vi "Locate Table.vi"(8 "error in":errorcluster, 11 "picture":refnum<vi>) -> (0 "error out":errorcluster, 3 "T":T1 format="%.3f", 5 "picture":picture)   [LabVIEW 2013]
uses:
  <vilib>/Analysis/Matrix/Datatypes/RealMatrix.ctl
  ROS/Code/SubVIs/BaxterSide.ctl
  <vilib>/Analysis/baseanly.llb/Mean (DBL).vi
  Baxter Examples/Arm Globals.vi
  Move/Move XYZOAT.vi
  Move/Move Axis.vi
  <vilib>/Analysis/baseanly.llb/Real Inverse Matrix.vi
  Prim/Fwd Kenimatics - array.vi
  <vilib>/Analysis/Matrix/Numeric/Multiply/Multiply - RM,RM.vi
  <vilib>/Analysis/Matrix/NI_Matrix.lvlib
  <vilib>/Analysis/NI_AALBase.lvlib
panel:
  out "Range":dbl
  out "result":cluster{"x":dbl, "y":dbl, "a":dbl}
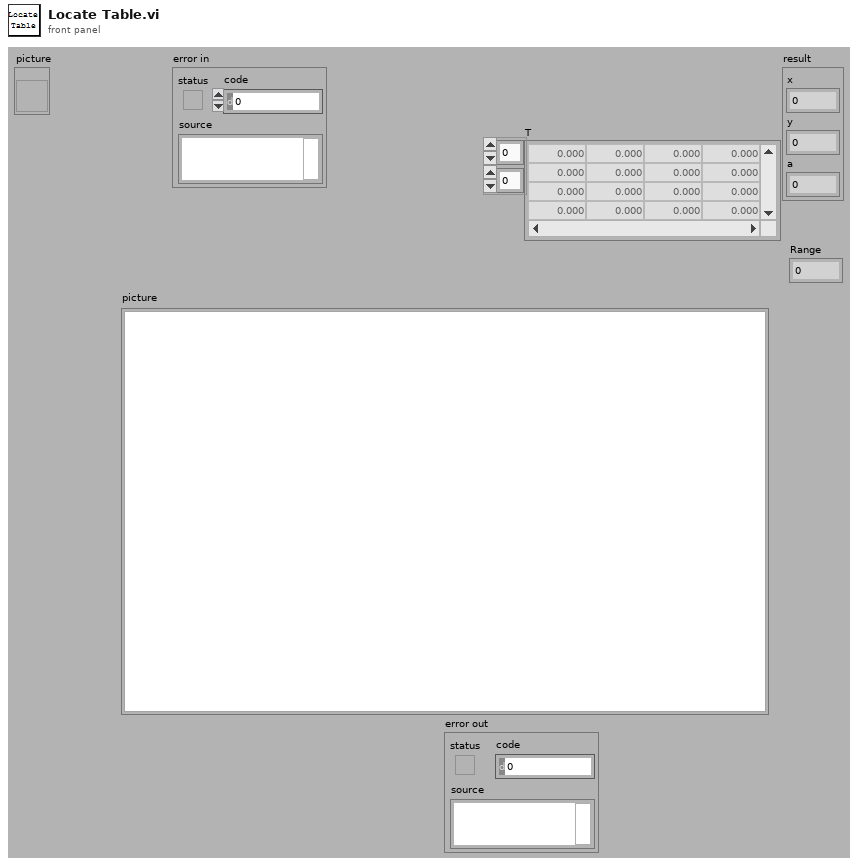
[diagram p1: front panel]
types:
  T1 = typedef "NI_Matrix.lvlib/RealMatrix.ctl" = dbl[][]
  T2 = typedef "BaxterSide.ctl" = enum16{"left", "right"}
  T3 = cluster{"Label":string, "Joints":dbl[], "T":T1}[]
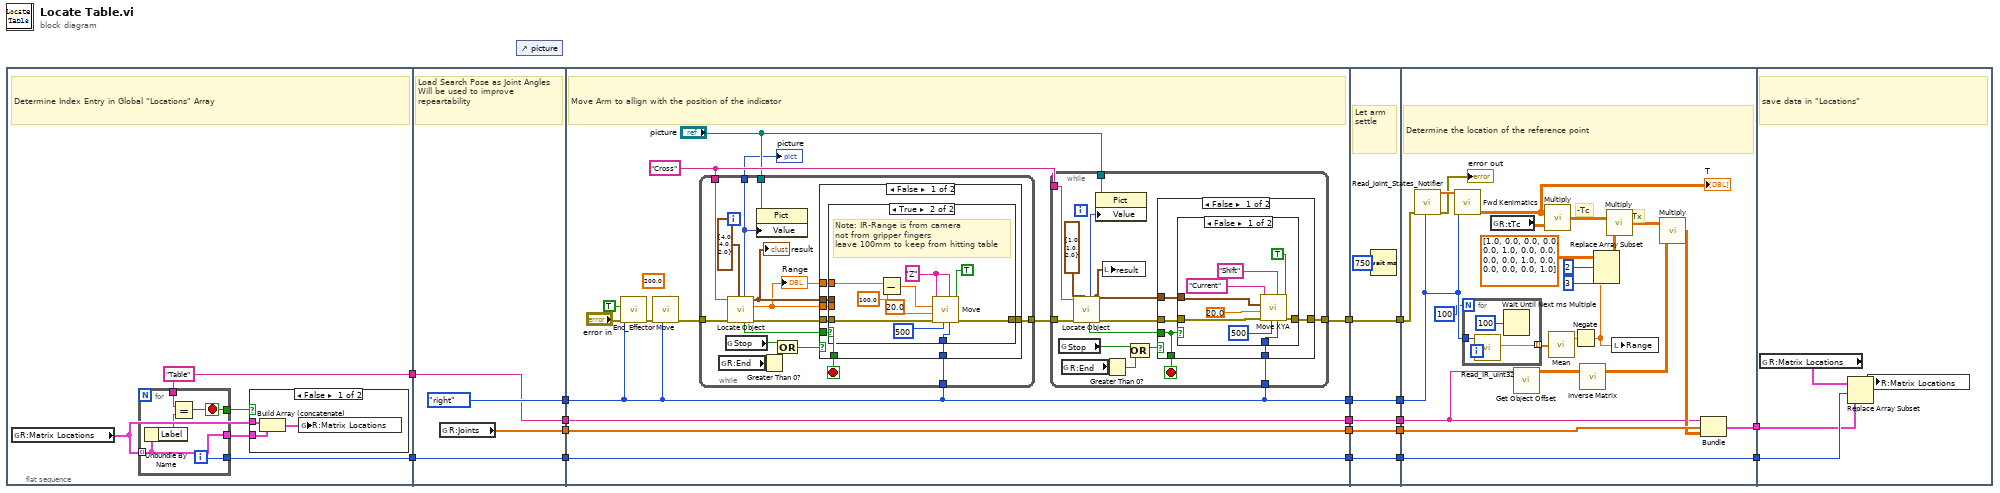
[diagram p0: block diagram]
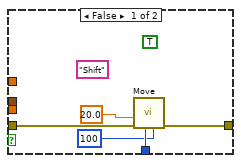
[diagram p5: hidden frame]
diagram:
  n1 = flat-sequence {
    tunnel: [w21] -> w11
    tunnel: [w23] -> w6
    tunnel: [BaxterSide."right" ("Side")] -> w14
    tunnel: [w32] -> w13
    tunnel: [w34] -> w12
    tunnel: w11 -> [w34]
    tunnel: [w33] -> w7
    tunnel: w6 -> [w33]
    tunnel: [w40] -> w17
    tunnel: [w42] -> w15
    tunnel: w14 -> [w40]
    tunnel: w13 -> [w38]
    tunnel: w12 -> [w37]
    tunnel: [w38] -> w10
    tunnel: [w37] -> w9
    tunnel: [w36] -> w8
    tunnel: w7 -> [w36]
    tunnel: [w125] -> w18
    tunnel: w17 -> [w125]
    tunnel: [w124] -> w16
    tunnel: w15 -> [w124]
    tunnel: w10 -> [w122]
    tunnel: w9 -> [w121]
    tunnel: w8 -> [w123]
    tunnel: [w123] -> w5
    tunnel: [w122] -> w4
    tunnel: [w121] -> w2
    tunnel: w18 -> [w139]
    tunnel: w16 -> [w147]
    tunnel: w5 -> [w131]
    tunnel: w4 -> [w134]
    tunnel: [w135] -> w3
    tunnel: w2 -> [w135]
    tunnel: [w132] -> w1
    tunnel: w3 -> [w154]
    tunnel: w1 -> [w153]
    frame #0 {
      w23 = "Table"
      # "Determine Index Entry in Global \"Locations\" Array"
      n2 = global read "Arm Globals.vi" "R:Matrix Locations"() -> (w19:T3)
      n3 = for {
        tunnel: w19 -> [w27] mode=indexing
        tunnel: w23 -> [w31]
        tunnel: [w30] -> w21
        tunnel: [w29] -> w22
        tunnel: [w27] -> w20
        i -> [w30]
        stop <- w29 stop-if-true
        n4 = Unbundle By Name(w27) -> ("Label"=w28:string)
        n5 = Equal?(x=w31, y=w28) -> (x = y?=w29:bool)
      }
      n6 = case shown="False" w22 {
        tunnel: w20 -> [w26 _]
        tunnel: w19 -> [w24 _]
        frame False {
          n7 = Build Array (concatenate)(w24, w26) -> (w25:T3)
          n8 = global write "Arm Globals.vi" "R:Matrix Locations"(w25) -> ()
        }
        frame True {
        }
      }
    }
    frame #1 {
      # "Load Search Pose as Joint Angles\nWill be used to improve repeartability"
      n9 = global read "Arm Globals.vi" "R:Joints"() -> (w32:dbl[])
    }
    frame #2 {
      (unwired) 200.0 ("Z")
      w44 = "Cross"
      # "Move Arm to allign with the position of the indicator"
      n10 = call "End_Effector.vi"("error in"="error in", "Close"=TRUE, "Side"=w40) -> ("error out"=w46:errorcluster)  [unwired: 5 in]
      n11 = call-poly "Move.vi"("Wait Time"=w40, "error in"=w46) -> ("error out"=w45:errorcluster)  [unwired: 9 in]
      n12 = while {
        tunnel: w45 -> [w96]
        tunnel: [w94] -> w48
        tunnel: w44 -> [w91]
        tunnel: w40 -> [w90]
        tunnel: "picture" -> [w85]
        tunnel: [w83] -> w39
        stop <- w88 stop-if-true
        n13 = global read "Arm Globals.vi" "R:End"() -> (w86:i32)
        n14 = global read "Arm Globals.vi" "Stop"() -> (w92:bool)
        n15 = call "Locate Object.vi"("Tolerance"=cluster{"x":dbl, "y":dbl, "a":dbl} {"x"=4.0, "y"=4.0, "a"=2.0}, "error in"=w96, "Object"=w91) -> ("error out"=w95:errorcluster, "Range"=w82:dbl, "result"=w93:cluster{"x":dbl, "y":dbl, "a":dbl}, "Close"=w87:bool, "picture"=w83:picture)  [unwired: 3 in, 1 out]
        "result" <- w93
        "Range" <- w82
        n16 = property class="Pict"(reference=w85, "Value"=w83) -> ()  [unwired: 1 in, 2 out]
        n17 = Greater Than 0?(x=w86) -> (x > 0?=w81:bool)
        n18 = Compound Arithmetic op=OR(w92, w81) -> (w89:bool)
        n19 = case shown="False" w89 {
          selector: w89 -> [_ w119]
          tunnel: w95 -> [w103 w120]
          tunnel: [w102 w120] -> w94
          tunnel: w93 -> [w101 _]
          tunnel: w90 -> [w100 _]
          tunnel: [w99 w119] -> w88
          tunnel: w87 -> [w99 _]
          tunnel: w82 -> [w98 _]
          tunnel: w82 -> [w97 _]
          frame False {
            n20 = case shown="True" w99 {
              tunnel: w103 -> [w108 w118]
              tunnel: [w107 w117] -> w102
              tunnel: w101 -> [_ _]
              tunnel: w100 -> [w106 w109]
              tunnel: w98 -> [_ _]
              tunnel: w97 -> [_ w115]
              frame False {
                (unwired) "Shift" ("Label")
                (unwired) TRUE ("Make Vertical")
                n21 = call-poly "Move.vi"("Side"=100 ("wait time"), "Wait Time"=w106, "error in"=w108, "Speed (mm/s)"=20.0) -> ("error out"=w107:errorcluster)  [unwired: 7 in]
              }
              frame True {
                w112 = "Z" ("Label")
                # "Note: IR-Range is from camera \nnot from gripper fingers\nleave 100mm to keep from hitting table"
                n22 = Subtract(x=w115, y=100.0) -> (x-y=w111:dbl)
                n23 = call-poly "Move.vi"("Make Vertical"=TRUE, "Side"=w109, "Label"=w112, "Wait Time"=500 ("wait time"), "error in"=w118, "Speed"=20.0, "Value"=w111, "Location"=w112) -> ("error out"=w117:errorcluster)  [unwired: 3 in]
              }
            }
          }
          frame True {
          }
        }
      }
      "picture" <- w39
      n24 = while {
        tunnel: w48 -> [w63]
        tunnel: [w61] -> w42
        tunnel: w44 -> [w58]
        tunnel: w40 -> [w57]
        tunnel: "picture" -> [w52]
        stop <- w54 stop-if-true
        n25 = global read "Arm Globals.vi" "Stop"() -> (w59:bool)
        n26 = global read "Arm Globals.vi" "R:End"() -> (w53:i32)
        n27 = call "Locate Object.vi"("Tolerance"=cluster{"x":dbl, "y":dbl, "a":dbl} {"x"=1.0, "y"=1.0, "a"=2.0}, "error in"=w63, "Object"=w58) -> ("error out"=w62:errorcluster, "result"=w60:cluster{"x":dbl, "y":dbl, "a":dbl}, "Close"=w55:bool, "picture"=w51:picture)  [unwired: 3 in, 2 out]
        n28 = property class="Pict"(reference=w52, "Value"=w51) -> ()  [unwired: 1 in, 2 out]
        n29 = local write "result"(w60) -> ()
        n30 = Greater Than 0?(x=w53) -> (x > 0?=w49:bool)
        n31 = Compound Arithmetic op=OR(w59, w49) -> (w56:bool)
        n32 = case shown="False" w56 {
          selector: w56 -> [_ w79]
          tunnel: w55 -> [w64 _]
          tunnel: w62 -> [w68 w80]
          tunnel: [w67 w80] -> w61
          tunnel: w60 -> [w66 _]
          tunnel: w57 -> [w65 _]
          tunnel: [w64 w79] -> w54
          frame False {
            n33 = case shown="False" w64 {
              tunnel: w68 -> [w76 w78]
              tunnel: [w77 w78] -> w67
              tunnel: w66 -> [w71 _]
              tunnel: w65 -> [w70 _]
              frame False {
                n34 = call "Move XYA.vi"("Make Vertical"=TRUE, "Side"=w70, "Label"="Shift", "Wait Time"=500 ("wait time"), "error in"=w76, "Speed (mm/s)"=20.0 ("Speed"), "XYA"=w71, "Location"="Current" ("Label")) -> ("error out"=w77:errorcluster)  [unwired: 3 in]
              }
              frame True {
              }
            }
          }
          frame True {
          }
        }
      }
    }
    frame #3 {
      # "Let arm settle"
      n35 = Wait (ms)(milliseconds to wait=u32 750) -> ()  [unwired: 1 out]
    }
    frame #4 {
      # "-Tx"
      # "-Tc"
      # "Determine the location of the reference point"
      n36 = call "Read_Joint_States_Notifier.vi"("Side"=w139, "error in"=w147) -> ("error out"=→"error out":errorcluster, "Positions"=w149:dbl[])  [unwired: 5 in]
      n37 = call-poly "Fwd Kenimatics.vi"("Side"=w139, "Joints"=w149) -> ("Matrix"=w138:T1)  [unwired: 8 in, 1 out]
      "T" <- w138
      n38 = for {
        N: 100 -> [_]
        tunnel: w139 -> [w152]
        tunnel: [w151] -> w136 mode=indexing
        n39 = call "Read_IR_uint32.vi"("Side"=w152) -> ("Distance"=w151:dbl)  [unwired: 4 in, 3 out]
        n40 = Wait Until Next ms Multiple(millisecond multiple=u32 100) -> ()  [unwired: 1 out]
      }
      n41 = global read "Arm Globals.vi" "R:tTc"() -> (w146:T1)
      n42 = call "Get Object Offset.vi"("Label"=w131) -> ("T"=w130:T1)  [unwired: 7 in, 3 out]
      n43 = call-poly <vilib>:"Multiply.vi"("Real Matrix B"=w146, "Real Matrix A"=w138) -> ("A * B"=w142:T1)
      n44 = call-poly <vilib>:"Mean.vi"("X"=w136) -> ("mean"=w128:dbl)  [unwired: 1 out]
      n45 = Negate(x=w128) -> (-x=w127:dbl)
      n46 = call-poly <vilib>:"Inverse Matrix.vi"("Input Matrix"=w130) -> ("Inverse Matrix"=w140:T1)  [unwired: 1 in, 1 out]
      n47 = Replace Array Subset(array=T1 [[1.0, 0.0, 0.0, 0.0], [0.0, 1.0, 0.0, 0.0], [0.0, 0.0, 1.0, 0.0], [0.0, 0.0, 0.0, 1.0]] ("-Tw"), new element=w127, index (row)=2 ("disabled index (row)"), index (col)=3 ("disabled index (col)")) -> (w141:T1)
      n48 = call-poly <vilib>:"Multiply.vi"("Real Matrix B"=w141, "Real Matrix A"=w142) -> ("A * B"=w137:T1)
      n49 = local write "Range"(w127) -> ()
      n50 = call-poly <vilib>:"Multiply.vi"("Real Matrix B"=w140, "Real Matrix A"=w137) -> ("A * B"=w133:T1)
      n51 = Bundle(w131, "R:Joints"=w134, "A * B"=w133) -> (w132:cluster{string, "R:Joints":dbl[], "A * B":T1})  [unwired: 1 in]
    }
    frame #5 {
      # "save data in \"Locations\""
      n52 = global read "Arm Globals.vi" "R:Matrix Locations"() -> (w156:T3)
      n53 = Replace Array Subset(array=w156, new element=w153, index=w154) -> (w155:T3)
      n54 = global write "Arm Globals.vi" "R:Matrix Locations"(w155) -> ()
    }
  }
  n55 = control-ref of="picture"() -> ()  [unwired: 1 out]
